vi "map_XY_stiffback.vi"() -> ()   [LabVIEW 2015]
panel:
  out "Mapping XY Stiffback":string
  in  "zero z":bool
  in  "ZeroLaser":bool
  in  "Done":bool
  in  "z down":bool
  in  "START MEASUREMENT":bool
  in  "KILL":bool
  in  "PAUSE":bool
  in  "RESUME":bool
  in  "QUIT":bool
  in  "Done":bool
  in  "z go to reading distance":bool
  in  "x go to stiffback":bool
  in  "y go to stiffback":bool
  in  "End":bool
  in  "zero z - end":bool
  in  "zero x - end":bool
  in  "zero y - end":bool
  out "output":string
  out "command":string
  in  "zero done":bool
  in  "zero z":bool
  in  "zero x":bool
  in  "zero y":bool
  # "Comandi di emergenza"
  # "MAPPING XY STIFFBACK"
  # "Posiziono in zero"
  # "Vado giu' ed azzero sul\nmarmo e rivado a zero\nin z"
  # "Vado sulla piastra \nsul primo punto"
  # "Ritorno a zero"
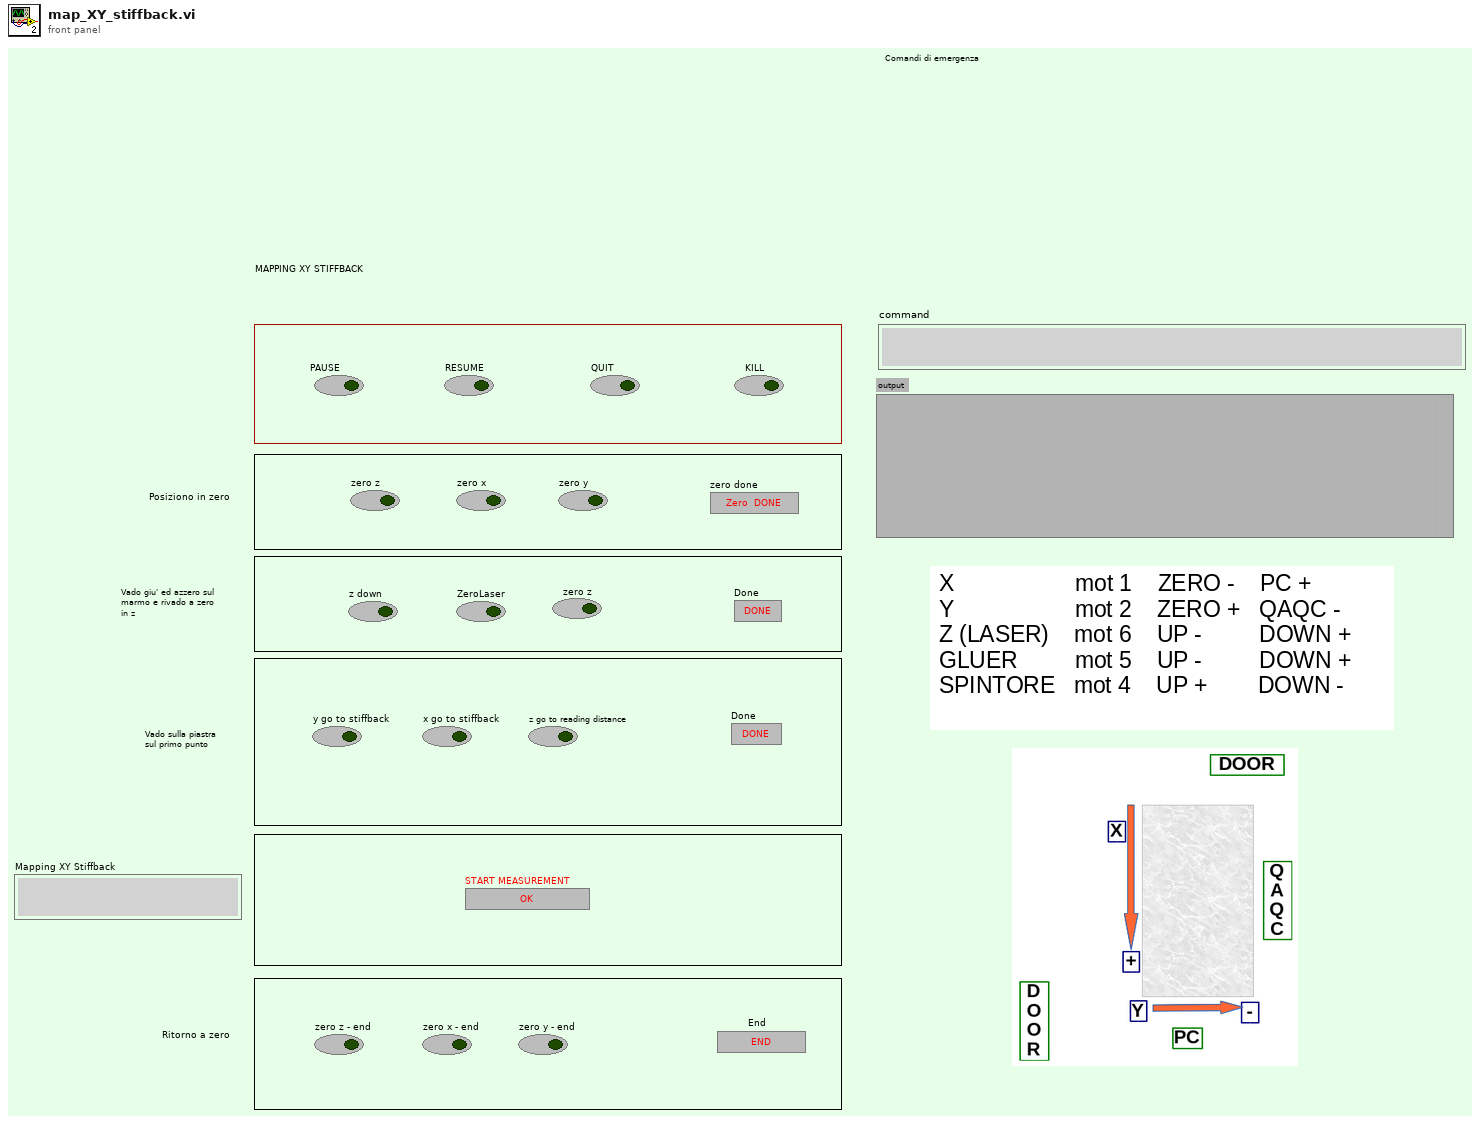
[diagram p1: front panel]
types:
  T1 = enum16{"open", "replace", "create", "open or create", "replace or create", "replace or create with confirmation"}
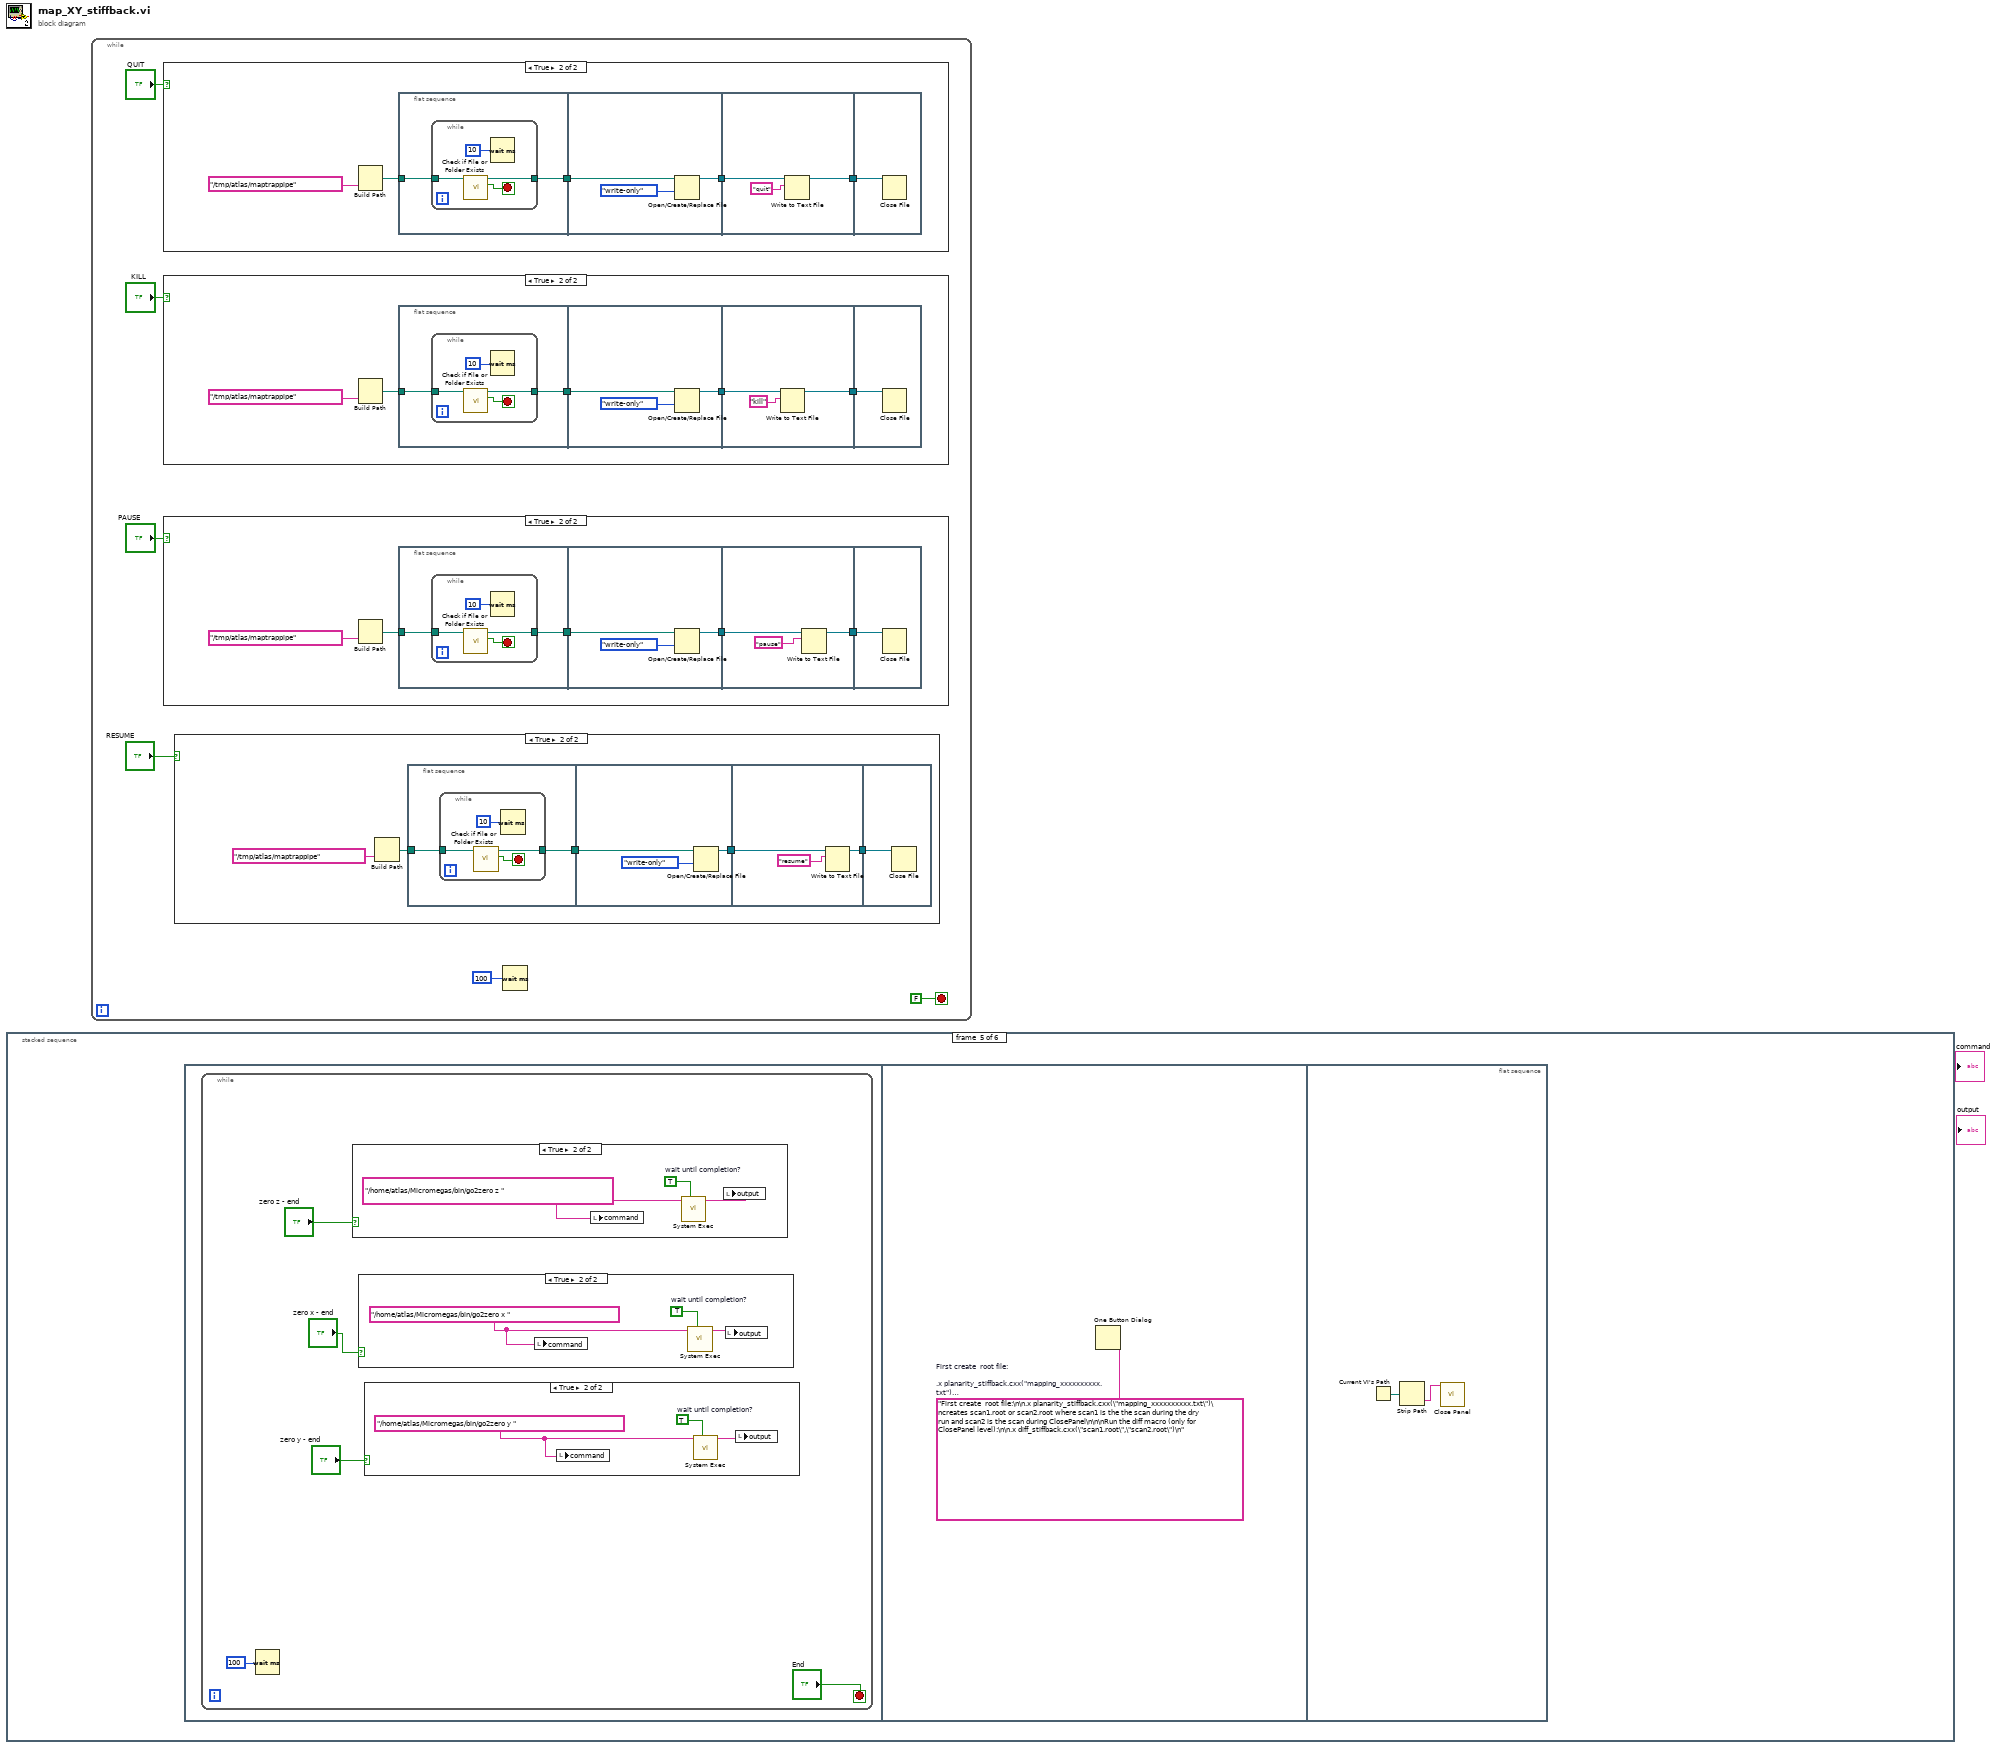
[diagram p0: block diagram]
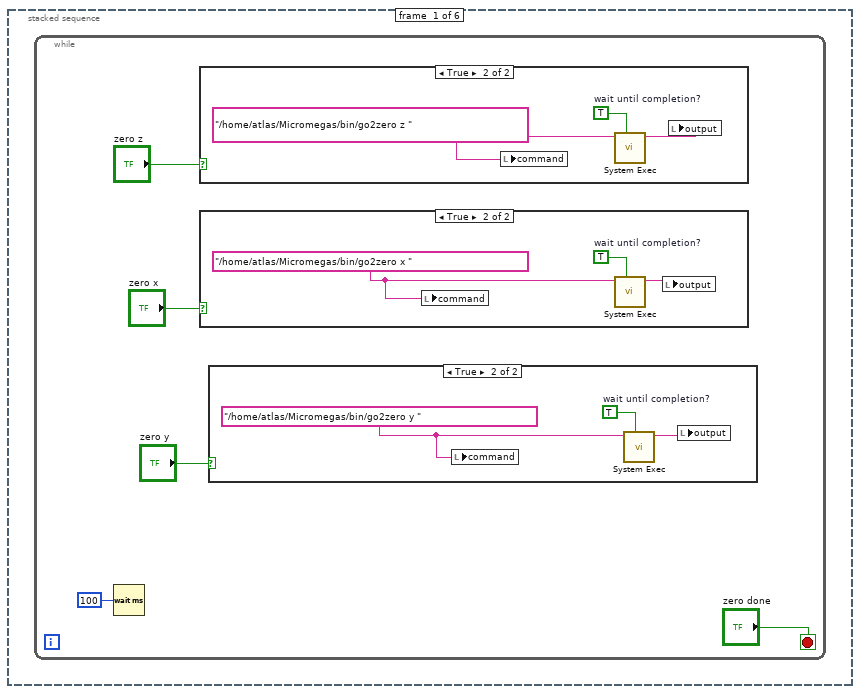
[diagram p6: hidden frame]
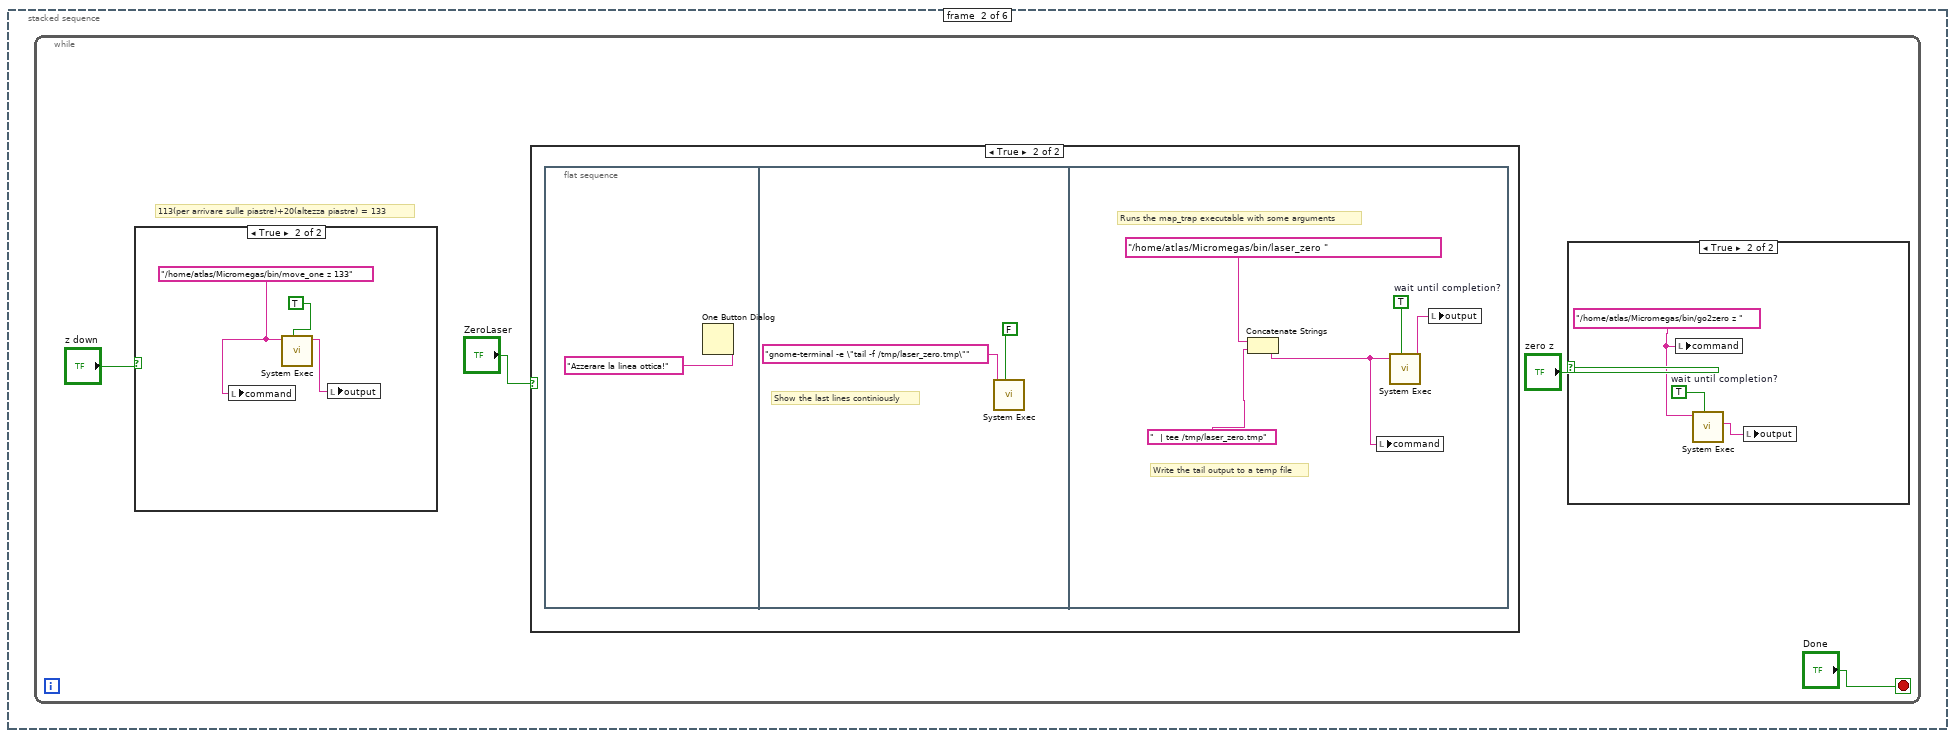
[diagram p10: hidden frame]
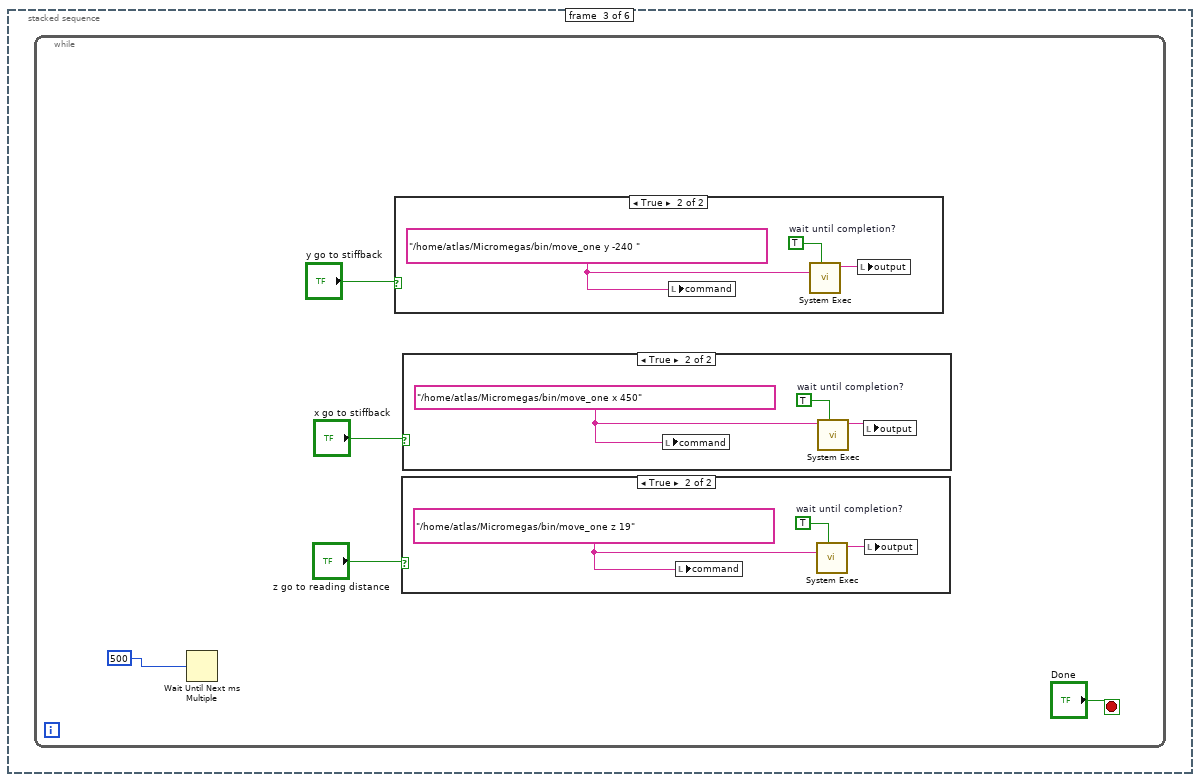
[diagram p14: hidden frame]
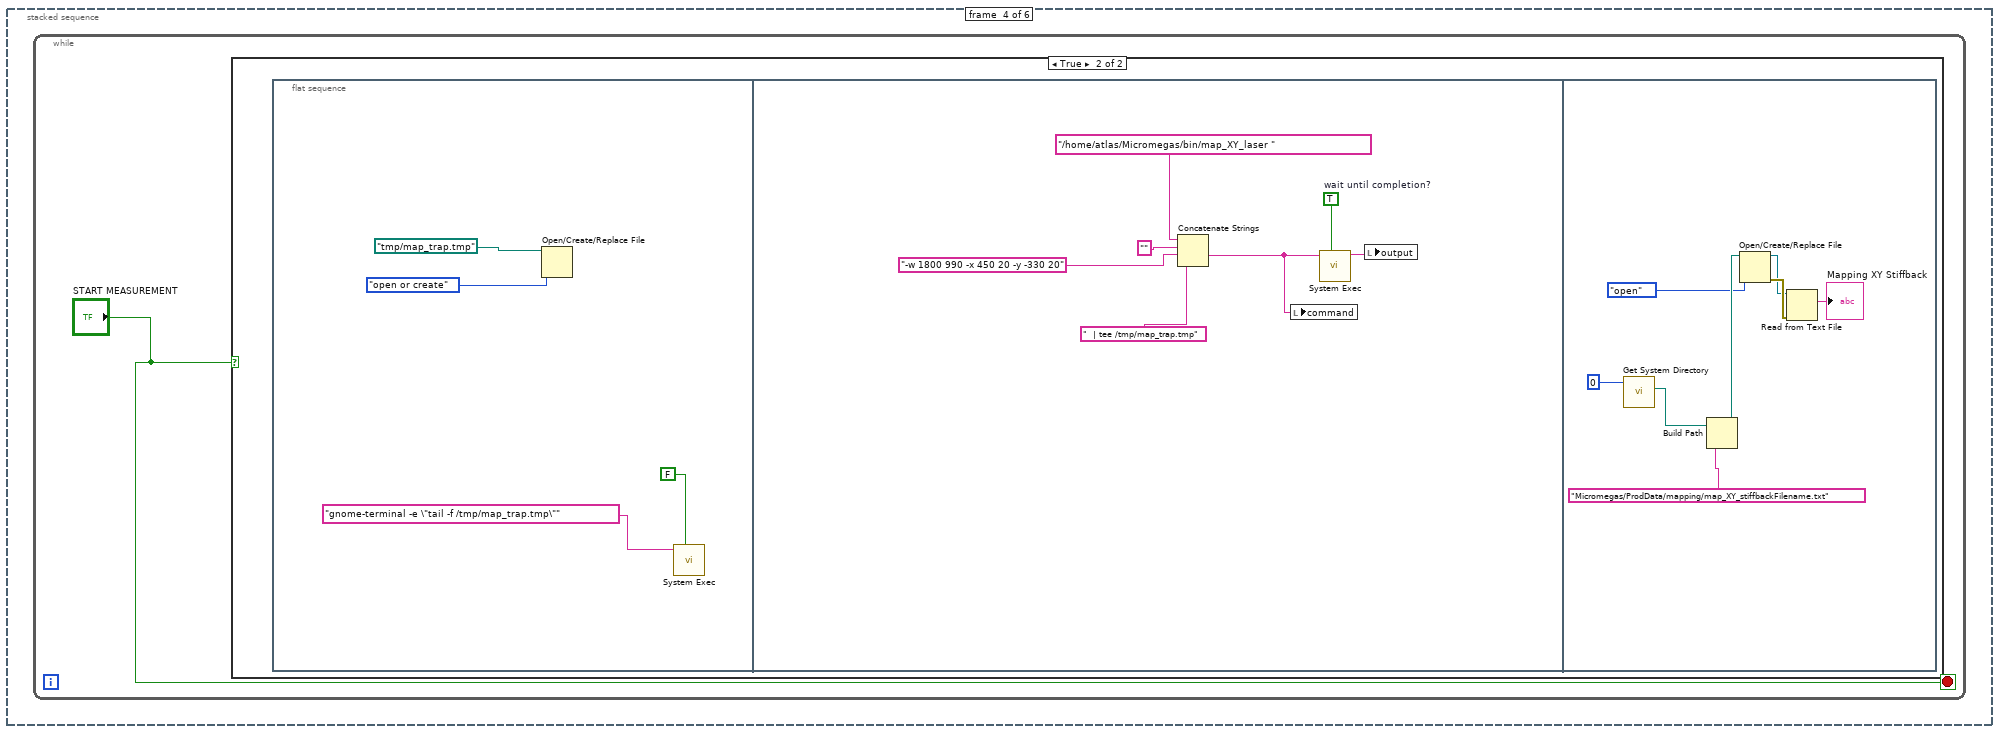
[diagram p18: hidden frame]
diagram:
  n1 = stacked-sequence {
    frame #0 {
      n2 = while {
        stop <- "zero done" stop-if-true
        n3 = Wait (ms)(milliseconds to wait=u32 100) -> ()  [unwired: 1 out]
        n4 = case shown="True" "zero z" {
          frame False {
          }
          frame True {
            w13 = "/home/atlas/Micromegas/bin/go2zero z " ("string")
            w14 = TRUE  # wait until completion?
            n5 = local write "command"(w13) -> ()
            n6 = call <vilib>:"System Exec.vi"("wait until completion? (T)"=w14, "command line"=w13) -> ("standard output"=w12:string)  [unwired: 6 in, 3 out]
            n7 = local write "output"(w12) -> ()
          }
        }
        n8 = case shown="True" "zero x" {
          frame False {
          }
          frame True {
            w10 = "/home/atlas/Micromegas/bin/go2zero x " ("string")
            w11 = TRUE  # wait until completion?
            n9 = local write "command"(w10) -> ()
            n10 = call <vilib>:"System Exec.vi"("wait until completion? (T)"=w11, "command line"=w10) -> ("standard output"=w9:string)  [unwired: 6 in, 3 out]
            n11 = local write "output"(w9) -> ()
          }
        }
        n12 = case shown="True" "zero y" {
          frame False {
          }
          frame True {
            w7 = "/home/atlas/Micromegas/bin/go2zero y " ("string")
            w8 = TRUE  # wait until completion?
            n13 = local write "command"(w7) -> ()
            n14 = call <vilib>:"System Exec.vi"("wait until completion? (T)"=w8, "command line"=w7) -> ("standard output"=w6:string)  [unwired: 6 in, 3 out]
            n15 = local write "output"(w6) -> ()
          }
        }
      }
    }
    frame #1 {
      n16 = while {
        stop <- "Done" stop-if-true
        # "113(per arrivare sulle piastre)+20(altezza piastre) = 133"
        n17 = case shown="True" "z down" {
          frame False {
          }
          frame True {
            w23 = "/home/atlas/Micromegas/bin/move_one z 133"
            n18 = local write "command"(w23) -> ()
            n19 = call <vilib>:"System Exec.vi"("wait until completion? (T)"=TRUE, "command line"=w23) -> ("standard output"=w22:string)  [unwired: 6 in, 3 out]
            n20 = local write "output"(w22) -> ()
          }
        }
        n21 = case shown="True" "ZeroLaser" {
          frame False {
          }
          frame True {
            n22 = flat-sequence {
              frame #0 {
                n23 = One Button Dialog(message="Azzerare la linea ottica!") -> ()  [unwired: 1 in, 1 out]
              }
              frame #1 {
                # "Show the last lines continiously"
                n24 = call <vilib>:"System Exec.vi"("wait until completion? (T)"=FALSE, "command line"="gnome-terminal -e \"tail -f /tmp/laser_zero.tmp\"") -> ()  [unwired: 6 in, 4 out]
              }
              frame #2 {
                w32 = TRUE  # wait until completion?
                # "Write the tail output to a temp file"
                # "Runs the map_trap executable with some arguments"
                n25 = Concatenate Strings("/home/atlas/Micromegas/bin/laser_zero " ("string"), "  | tee /tmp/laser_zero.tmp" ("string")) -> (w28:string)
                n26 = local write "command"(w28) -> ()
                n27 = call <vilib>:"System Exec.vi"("wait until completion? (T)"=w32, "command line"=w28) -> ("standard output"=w29:string)  [unwired: 6 in, 3 out]
                n28 = local write "output"(w29) -> ()
              }
            }
          }
        }
        n29 = case shown="True" "zero z" {
          frame False {
          }
          frame True {
            w21 = TRUE  # wait until completion?
            w19 = "/home/atlas/Micromegas/bin/go2zero z " ("string")
            n30 = local write "command"(w19) -> ()
            n31 = call <vilib>:"System Exec.vi"("wait until completion? (T)"=w21, "command line"=w19) -> ("standard error"=w20:string)  [unwired: 6 in, 3 out]
            n32 = local write "output"(w20) -> ()
          }
        }
      }
    }
    frame #2 {
      n33 = while {
        stop <- "Done" stop-if-true
        n34 = Wait Until Next ms Multiple(millisecond multiple=u32 500 ("millisecond timer value")) -> ()  [unwired: 1 out]
        n35 = case shown="True" "y go to stiffback" {
          frame False {
          }
          frame True {
            w44 = "/home/atlas/Micromegas/bin/move_one y -240 " ("string")
            w46 = TRUE  # wait until completion?
            n36 = local write "command"(w44) -> ()
            n37 = call <vilib>:"System Exec.vi"("wait until completion? (T)"=w46, "command line"=w44) -> ("standard output"=w45:string)  [unwired: 6 in, 3 out]
            n38 = local write "output"(w45) -> ()
          }
        }
        n39 = case shown="True" "z go to reading distance" {
          frame False {
          }
          frame True {
            w38 = "/home/atlas/Micromegas/bin/move_one z 19" ("string")
            w40 = TRUE  # wait until completion?
            n40 = local write "command"(w38) -> ()
            n41 = call <vilib>:"System Exec.vi"("wait until completion? (T)"=w40, "command line"=w38) -> ("standard output"=w39:string)  [unwired: 6 in, 3 out]
            n42 = local write "output"(w39) -> ()
          }
        }
        n43 = case shown="True" "x go to stiffback" {
          frame False {
          }
          frame True {
            w41 = "/home/atlas/Micromegas/bin/move_one x 450" ("string")
            w43 = TRUE  # wait until completion?
            n44 = local write "command"(w41) -> ()
            n45 = call <vilib>:"System Exec.vi"("wait until completion? (T)"=w43, "command line"=w41) -> ("standard output"=w42:string)  [unwired: 6 in, 3 out]
            n46 = local write "output"(w42) -> ()
          }
        }
      }
    }
    frame #3 {
      n47 = while {
        stop <- "START MEASUREMENT" stop-if-true
        n48 = case shown="True" "START MEASUREMENT" {
          frame False {
          }
          frame True {
            n49 = flat-sequence {
              frame #0 {
                n50 = Open/Create/Replace File(file path (use dialog)=path "/tmp/map_trap.tmp", operation (0:open)=T1."open or create") -> ()  [unwired: 4 in, 3 out]
                n51 = call <vilib>:"System Exec.vi"("wait until completion? (T)"=FALSE, "command line"="gnome-terminal -e \"tail -f /tmp/map_trap.tmp\"") -> ()  [unwired: 6 in, 4 out]
              }
              frame #1 {
                w58 = TRUE  # wait until completion?
                n52 = Concatenate Strings("/home/atlas/Micromegas/bin/map_XY_laser " ("string"), "" ("string"), "-w 1800 990 -x 450 20 -y -330 20" ("string"), "  | tee /tmp/map_trap.tmp" ("string")) -> (w53:string)
                n53 = local write "command"(w53) -> ()
                n54 = call <vilib>:"System Exec.vi"("wait until completion? (T)"=w58, "command line"=w53) -> ("standard output"=w52:string)  [unwired: 6 in, 3 out]
                n55 = local write "output"(w52) -> ()
              }
              frame #2 {
                n56 = call <vilib>:"Get System Directory.vi"("system directory type"=0) -> ("system directory"=w65:path)  [unwired: 10 in]
                n57 = Build Path(base path=w65, name or relative path="Micromegas/ProdData/mapping/map_XY_stiffbackFilename.txt") -> (appended path=w66:path)
                n58 = Open/Create/Replace File(file path (use dialog)=w66, operation (0:open)=T1."open") -> (refnum out=w60:refnum<file>, error out=w61:errorcluster)  [unwired: 4 in, 1 out]
                n59 = Read from Text File(file (use dialog)=w60, error in=w61) -> (text=→"Mapping XY Stiffback":string)  [unwired: 2 in, 3 out]
              }
            }
          }
        }
      }
    }
    frame #4 {
      n60 = flat-sequence {
        frame #0 {
          n61 = while {
            stop <- "End" stop-if-true
            n62 = Wait (ms)(milliseconds to wait=u32 100) -> ()  [unwired: 1 out]
            n63 = case shown="True" "zero z - end" {
              frame False {
              }
              frame True {
                w79 = "/home/atlas/Micromegas/bin/go2zero z " ("string")
                w80 = TRUE  # wait until completion?
                n64 = local write "command"(w79) -> ()
                n65 = call <vilib>:"System Exec.vi"("wait until completion? (T)"=w80, "command line"=w79) -> ("standard output"=w78:string)  [unwired: 6 in, 3 out]
                n66 = local write "output"(w78) -> ()
              }
            }
            n67 = case shown="True" "zero x - end" {
              frame False {
              }
              frame True {
                w76 = "/home/atlas/Micromegas/bin/go2zero x " ("string")
                w77 = TRUE  # wait until completion?
                n68 = local write "command"(w76) -> ()
                n69 = call <vilib>:"System Exec.vi"("wait until completion? (T)"=w77, "command line"=w76) -> ("standard output"=w75:string)  [unwired: 6 in, 3 out]
                n70 = local write "output"(w75) -> ()
              }
            }
            n71 = case shown="True" "zero y - end" {
              frame False {
              }
              frame True {
                w73 = "/home/atlas/Micromegas/bin/go2zero y " ("string")
                w74 = TRUE  # wait until completion?
                n72 = local write "command"(w73) -> ()
                n73 = call <vilib>:"System Exec.vi"("wait until completion? (T)"=w74, "command line"=w73) -> ("standard output"=w72:string)  [unwired: 6 in, 3 out]
                n74 = local write "output"(w72) -> ()
              }
            }
          }
        }
        frame #1 {
          w81 = "First create  root file:\n\n.x planarity_stiffback.cxx(\"mapping_xxxxxxxxxx.txt\")\ncreates scan1.root or scan2.root where scan1 is the the scan during the dry run and scan2 is the scan during ClosePanel\n\n\nRun the diff macro (only for ClosePanel level):\n\n.x diff_stiffback.cxx(\"scan1.root\",\"scan2.root\")\n"  # First create  root file:  .x planarity_stiffback.cxx("mapping_xxxxxxxxxx.txt") creates scan1.root or scan2.root where scan1 is the the scan during the dry run and scan2 is the scan during ClosePanel   Run the diff macro (only for ClosePanel level):  .x diff_stiffback.cxx("scan1.root","scan2.root")
          n75 = One Button Dialog(message=w81) -> ()  [unwired: 1 in, 1 out]
        }
        frame #2 {
          n76 = Current VI's Path() -> (path=w83:path)
          n77 = Strip Path(path=w83) -> (name=w82:string)  [unwired: 1 out]
          n78 = call <vilib>:"Close Panel.vi"("VI name"=w82) -> ()  [unwired: 10 in, 1 out]
        }
      }
    }
    frame #5 {
      n79 = One Button Dialog(message="Per comodita`, rinominare il file (non verra` comunque sovrascritto)") -> ()  [unwired: 1 in, 1 out]
    }
  }
  n80 = while {
    stop <- FALSE stop-if-true
    n81 = case shown="True" "QUIT" {
      frame False {
      }
      frame True {
        n82 = Build Path(name or relative path="/tmp/atlas/maptrappipe" ("string")) -> (appended path=w145:path)  [unwired: 1 in]
        n83 = flat-sequence {
          tunnel: [w151] -> w149
          tunnel: w145 -> [w150]
          tunnel: w149 -> [w158]
          tunnel: [w156] -> w148
          tunnel: w148 -> [w161]
          tunnel: [w160] -> w147
          tunnel: w147 -> [w162]
          frame #0 {
            n84 = while {
              tunnel: [w153] -> w151
              tunnel: w150 -> [w152]
              stop <- w154 stop-if-true
              n85 = call <vilib>:"Check if File or Folder Exists.vi"("path"=w152) -> ("file or folder exists?"=w154:bool, "dup path"=w153:path)  [unwired: 8 in, 1 out]
              n86 = Wait (ms)(milliseconds to wait=u32 10) -> ()  [unwired: 1 out]
            }
          }
          frame #1 {
            n87 = Open/Create/Replace File(file path (use dialog)=w158, access (0:read/write)=enum16{"read/write", "read-only", "write-only"}."write-only") -> (refnum out=w156:refnum<file>)  [unwired: 4 in, 2 out]
          }
          frame #2 {
            n88 = Write to Text File(file (use dialog)=w161, text="quit") -> (refnum out=w160:refnum<file>)  [unwired: 2 in, 2 out]
          }
          frame #3 {
            n89 = Close File(refnum=w162) -> ()  [unwired: 1 in, 2 out]
          }
        }
      }
    }
    n90 = case shown="True" "KILL" {
      frame False {
      }
      frame True {
        n91 = Build Path(name or relative path="/tmp/atlas/maptrappipe" ("string")) -> (appended path=w109:path)  [unwired: 1 in]
        n92 = flat-sequence {
          tunnel: [w115] -> w113
          tunnel: w109 -> [w114]
          tunnel: w113 -> [w122]
          tunnel: [w120] -> w112
          tunnel: w112 -> [w125]
          tunnel: [w124] -> w111
          tunnel: w111 -> [w126]
          frame #0 {
            n93 = while {
              tunnel: [w117] -> w115
              tunnel: w114 -> [w116]
              stop <- w118 stop-if-true
              n94 = call <vilib>:"Check if File or Folder Exists.vi"("path"=w116) -> ("file or folder exists?"=w118:bool, "dup path"=w117:path)  [unwired: 8 in, 1 out]
              n95 = Wait (ms)(milliseconds to wait=u32 10) -> ()  [unwired: 1 out]
            }
          }
          frame #1 {
            n96 = Open/Create/Replace File(file path (use dialog)=w122, access (0:read/write)=enum16{"read/write", "read-only", "write-only"}."write-only") -> (refnum out=w120:refnum<file>)  [unwired: 4 in, 2 out]
          }
          frame #2 {
            n97 = Write to Text File(file (use dialog)=w125, text="kill") -> (refnum out=w124:refnum<file>)  [unwired: 2 in, 2 out]
          }
          frame #3 {
            n98 = Close File(refnum=w126) -> ()  [unwired: 1 in, 2 out]
          }
        }
      }
    }
    n99 = case shown="True" "PAUSE" {
      frame False {
      }
      frame True {
        n100 = Build Path(name or relative path="/tmp/atlas/maptrappipe" ("string")) -> (appended path=w91:path)  [unwired: 1 in]
        n101 = flat-sequence {
          tunnel: [w97] -> w95
          tunnel: w91 -> [w96]
          tunnel: w95 -> [w104]
          tunnel: [w102] -> w94
          tunnel: w94 -> [w107]
          tunnel: [w106] -> w93
          tunnel: w93 -> [w108]
          frame #0 {
            n102 = while {
              tunnel: [w99] -> w97
              tunnel: w96 -> [w98]
              stop <- w100 stop-if-true
              n103 = call <vilib>:"Check if File or Folder Exists.vi"("path"=w98) -> ("file or folder exists?"=w100:bool, "dup path"=w99:path)  [unwired: 8 in, 1 out]
              n104 = Wait (ms)(milliseconds to wait=u32 10) -> ()  [unwired: 1 out]
            }
          }
          frame #1 {
            n105 = Open/Create/Replace File(file path (use dialog)=w104, access (0:read/write)=enum16{"read/write", "read-only", "write-only"}."write-only") -> (refnum out=w102:refnum<file>)  [unwired: 4 in, 2 out]
          }
          frame #2 {
            n106 = Write to Text File(file (use dialog)=w107, text="pause") -> (refnum out=w106:refnum<file>)  [unwired: 2 in, 2 out]
          }
          frame #3 {
            n107 = Close File(refnum=w108) -> ()  [unwired: 1 in, 2 out]
          }
        }
      }
    }
    n108 = case shown="True" "RESUME" {
      frame False {
      }
      frame True {
        n109 = Build Path(name or relative path="/tmp/atlas/maptrappipe" ("string")) -> (appended path=w127:path)  [unwired: 1 in]
        n110 = flat-sequence {
          tunnel: [w133] -> w131
          tunnel: w127 -> [w132]
          tunnel: w131 -> [w140]
          tunnel: [w138] -> w130
          tunnel: w130 -> [w143]
          tunnel: [w142] -> w129
          tunnel: w129 -> [w144]
          frame #0 {
            n111 = while {
              tunnel: [w135] -> w133
              tunnel: w132 -> [w134]
              stop <- w136 stop-if-true
              n112 = call <vilib>:"Check if File or Folder Exists.vi"("path"=w134) -> ("file or folder exists?"=w136:bool, "dup path"=w135:path)  [unwired: 8 in, 1 out]
              n113 = Wait (ms)(milliseconds to wait=u32 10) -> ()  [unwired: 1 out]
            }
          }
          frame #1 {
            n114 = Open/Create/Replace File(file path (use dialog)=w140, access (0:read/write)=enum16{"read/write", "read-only", "write-only"}."write-only") -> (refnum out=w138:refnum<file>)  [unwired: 4 in, 2 out]
          }
          frame #2 {
            n115 = Write to Text File(file (use dialog)=w143, text="resume") -> (refnum out=w142:refnum<file>)  [unwired: 2 in, 2 out]
          }
          frame #3 {
            n116 = Close File(refnum=w144) -> ()  [unwired: 1 in, 2 out]
          }
        }
      }
    }
    n117 = Wait (ms)(milliseconds to wait=100) -> ()  [unwired: 1 out]
  }
